vi "Get second.vi"(9 "date time rec":T1) -> (1 "output variable":i32)   [LabVIEW 2018]
uses:
  <vilib>/Utility/miscctls.llb/LVDateTimeRec.ctl
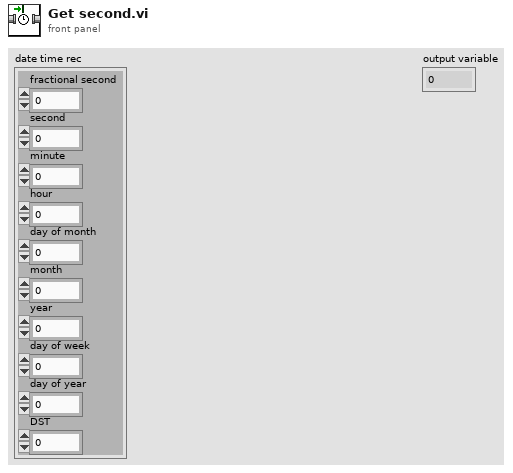
[diagram p1: front panel]
types:
  T1 = typedef "LVDateTimeRec.ctl" = cluster{"fractional second":dbl, "second":i32, "minute":i32, "hour":i32, "day of month":i32, "month":i32, "year":i32, "day of week":i32, "day of year":i32, "DST":i32}
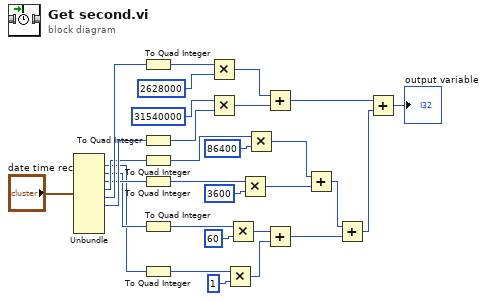
[diagram p0: block diagram]
diagram:
  n1 = Unbundle("date time rec") -> ("second"=w15:i32, "minute"=w16:i32, "hour"=w17:i32, "day of month"=w18:i32, "month"=w29:i32, "year"=w19:i32)  [unwired: 4 out]
  n2 = To Quad Integer(1:w29) -> (0:w28:i64)
  n3 = To Quad Integer(1:w19) -> (0:w25:i64)
  n4 = To Quad Integer(1:w18) -> (0:w23:i64)
  n5 = To Quad Integer(1:w17) -> (0:w21:i64)
  n6 = To Quad Integer(1:w16) -> (0:w11:i64)
  n7 = To Quad Integer(1:w15) -> (0:w12:i64)
  n8 = Multiply(x=w28, y=i64 2628000) -> (x*y=w26:i64)
  n9 = Multiply(x=i64 31540000, y=w25) -> (x*y=w10:i64)
  n10 = Multiply(x=w12, y=i64 1) -> (x*y=w5:i64)
  n11 = Multiply(x=w11, y=i64 60) -> (x*y=w6:i64)
  n12 = Multiply(x=w21, y=i64 3600) -> (x*y=w7:i64)
  n13 = Multiply(x=w23, y=i64 86400) -> (x*y=w8:i64)
  n14 = Add(x=w26, y=w10) -> (x+y=w9:i64)
  n15 = Add(x=w6, y=w5) -> (x+y=w4:i64)
  n16 = Add(x=w8, y=w7) -> (x+y=w3:i64)
  n17 = Add(x=w3, y=w4) -> (x+y=w2:i64)
  n18 = Add(x=w9, y=w2) -> (x+y=→"output variable":i64)
